vi "Sequence.InitializeChannel.vi"(8 "error in (no error)":errorcluster, 10 "ChannelName":string, 11 ".NET Refnum in":refnum<k24>) -> (0 "error out":errorcluster, 3 ".NET Refnum out":refnum<k24>)   [LabVIEW 2013, in "Simple Sequence Tools - Editor.lvlib"]
uses:
  Simple Sequence Tools - Editor.lvlib
  NationalInstruments.VeriStand.RealTimeSequenceDefinitionApi
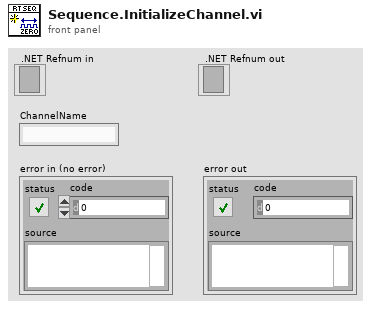
[diagram p1: front panel]
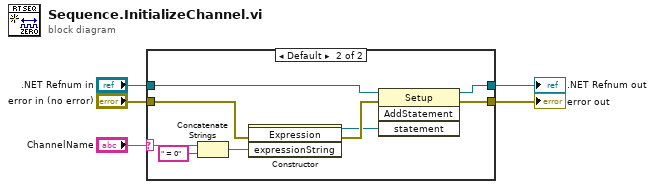
[diagram p0: block diagram]
diagram:
  n1 = case shown="Default" "ChannelName" {
    selector: "ChannelName" -> [_ w10]
    tunnel: "error in (no error)" -> [w7 w14]
    tunnel: [w7 w13] -> w2
    tunnel: ".NET Refnum in" -> [w6 w12]
    tunnel: [w6 w11] -> w4
    frame "" {
    }
    frame Default {
      n2 = Concatenate Strings(w10, " = 0" ("string")) -> (w8:string)
      n3 = constructor class="Expression"(error in=w14, "expressionString"=w8) -> (reference out=w15:refnum<k24>, error out=w16:errorcluster)  [unwired: 2 in, 2 out]
      n4 = invoke class="Setup" method="AddStatement"(reference=w12, error in=w16, "statement"=w15) -> (reference out=w11:refnum<k24>, error out=w13:errorcluster)  [unwired: 1 in, 2 out]
    }
  }
  ".NET Refnum out" <- w4
  "error out" <- w2
